vi "Calibration Range Lookup.vi"(9 "Samples To Collect":dbl, 10 "Temperature Units":T1 items=["Celcius", "Fahrenheit", "Kelvin", "Rankine"], 11 "Cal Channel TC Type":T2 items=["J", "K", "T", "E", "N", "B", "R", "S"]) -> (2 "X-axis Values":dbl[](array[numeric]))   [LabVIEW 2011, in "Simulated Thermocouple Custom Device.lvlib"]
uses:
  Simulated Thermocouple Custom Device.lvlib
  TC Selector.ctl
  TC Unit Selector.ctl
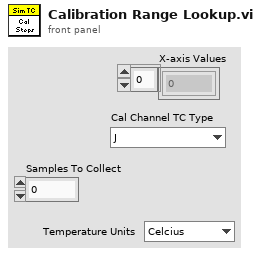
[diagram p1: front panel]
types:
  T1 = typedef "Simulated Thermocouple Custom Device.lvlib/TC Unit Selector.ctl" = u16
  T2 = typedef "Simulated Thermocouple Custom Device.lvlib/TC Selector.ctl" = u16
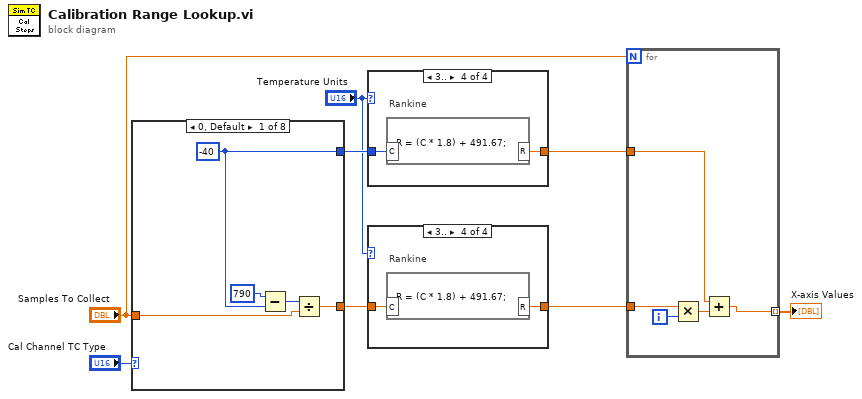
[diagram p0: block diagram]
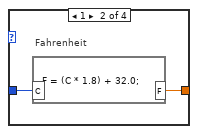
[diagram p3: hidden frame]
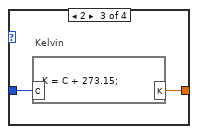
[diagram p4: hidden frame]
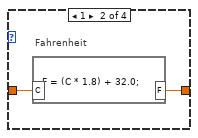
[diagram p6: hidden frame]
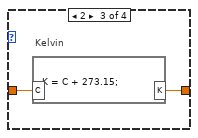
[diagram p7: hidden frame]
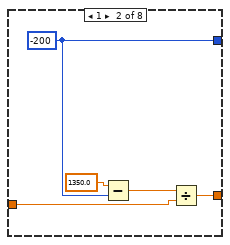
[diagram p8: hidden frame]
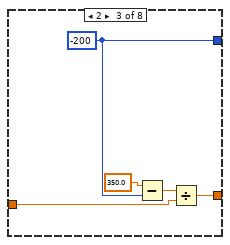
[diagram p9: hidden frame]
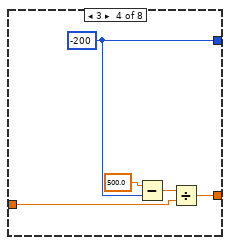
[diagram p10: hidden frame]
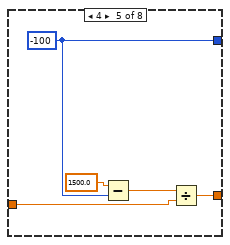
[diagram p11: hidden frame]
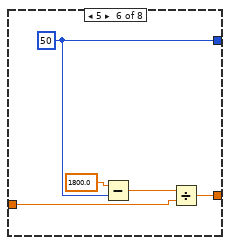
[diagram p12: hidden frame]
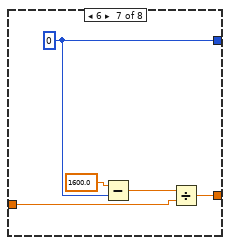
[diagram p13: hidden frame]
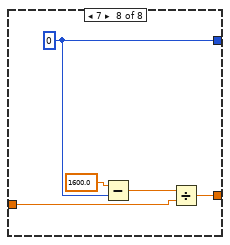
[diagram p14: hidden frame]
diagram:
  n1 = case shown="0, Default" "Cal Channel TC Type" {
    tunnel: "Samples To Collect" -> [w13 w17 w22 w27 w32 w37 w42 w47]
    tunnel: [w12 w18 w23 w28 w33 w38 w43 w48] -> w8
    tunnel: [w11 w14 w21 w26 w31 w35 w40 w46] -> w7
    frame 0, Default {
      w11 = -40
      n2 = Subtract(x=790, y=w11) -> (x-y=w9:i32)
      n3 = Divide(x=w9, y=w13) -> (x/y=w12:dbl)
    }
    frame 1 {
      w14 = -200
      n4 = Subtract(x=1350.0, y=w14) -> (x-y=w15:dbl)
      n5 = Divide(x=w15, y=w17) -> (x/y=w18:dbl)
    }
    frame 2 {
      w21 = -200
      n6 = Subtract(x=350.0, y=w21) -> (x-y=w19:dbl)
      n7 = Divide(x=w19, y=w22) -> (x/y=w23:dbl)
    }
    frame 3 {
      w26 = -200
      n8 = Subtract(x=500.0, y=w26) -> (x-y=w24:dbl)
      n9 = Divide(x=w24, y=w27) -> (x/y=w28:dbl)
    }
    frame 4 {
      w31 = -100
      n10 = Subtract(x=1500.0, y=w31) -> (x-y=w29:dbl)
      n11 = Divide(x=w29, y=w32) -> (x/y=w33:dbl)
    }
    frame 5 {
      w35 = 50
      n12 = Subtract(x=1800.0, y=w35) -> (x-y=w34:dbl)
      n13 = Divide(x=w34, y=w37) -> (x/y=w38:dbl)
    }
    frame 6 {
      w40 = 0
      n14 = Subtract(x=1600.0, y=w40) -> (x-y=w39:dbl)
      n15 = Divide(x=w39, y=w42) -> (x/y=w43:dbl)
    }
    frame 7 {
      w46 = 0
      n16 = Subtract(x=1600.0, y=w46) -> (x-y=w44:dbl)
      n17 = Divide(x=w44, y=w47) -> (x/y=w48:dbl)
    }
  }
  n18 = case shown="3.." "Temperature Units" {
    tunnel: [w49 w51 w53 w55] -> w6
    tunnel: w7 -> [w49 w50 w52 w54]
    frame ..0 {
      # "Celsius"
    }
    frame 1 {
      # "Fahrenheit"
      n19 = formula code="F = (C * 1.8) + 32.0;"("C"=w50) -> ("F"=w51:dbl)
    }
    frame 2 {
      # "Kelvin"
      n20 = formula code="K = C + 273.15;"("C"=w52) -> ("K"=w53:dbl)
    }
    frame 3.. {
      # "Rankine"
      n21 = formula code="R = (C * 1.8) + 491.67;"("C"=w54) -> ("R"=w55:dbl)
    }
  }
  n22 = case shown="3.." "Temperature Units" {
    tunnel: [w56 w58 w60 w62] -> w5
    tunnel: w8 -> [w56 w57 w59 w61]
    frame ..0 {
      # "Celsius"
    }
    frame 1 {
      # "Fahrenheit"
      n23 = formula code="F = (C * 1.8) + 32.0;"("C"=w57) -> ("F"=w58:dbl)
    }
    frame 2 {
      # "Kelvin"
      n24 = formula code="K = C + 273.15;"("C"=w59) -> ("K"=w60:dbl)
    }
    frame 3.. {
      # "Rankine"
      n25 = formula code="R = (C * 1.8) + 491.67;"("C"=w61) -> ("R"=w62:dbl)
    }
  }
  n26 = for {
    N: "Samples To Collect" -> [_]
    tunnel: w6 -> [w67]
    tunnel: w5 -> [w65]
    tunnel: [w63] -> w4 mode=indexing
    i -> [w66]
    n27 = Multiply(x=w65, y=w66) -> (x*y=w64:dbl)
    n28 = Add(x=w67, y=w64) -> (x+y=w63:dbl)
  }
  "X-axis Values" <- w4
